vi "VPA QC Try Get Old File Data.vi"(10 "Path (dialog)":path, 11 "State Data In":T4) -> (3 "State Cluster Out":T4)   [LabVIEW 2013]
uses:
  Controls/VPA QC State Data Cluster.ctl
  Controls/VPA QC General Cluster.ctl
  Controls/VPA QC State Enum.ctl
  Controls/VPA QC Bool Cluster.ctl
  Controls/VPA QC State Data Cluster Ver 4.ctl
panel:
  in  "State Cluster Ver  4":T1
  # "Assembly Checklist"
  # "Assembly Checklist"
  # "Assembly Checklist"
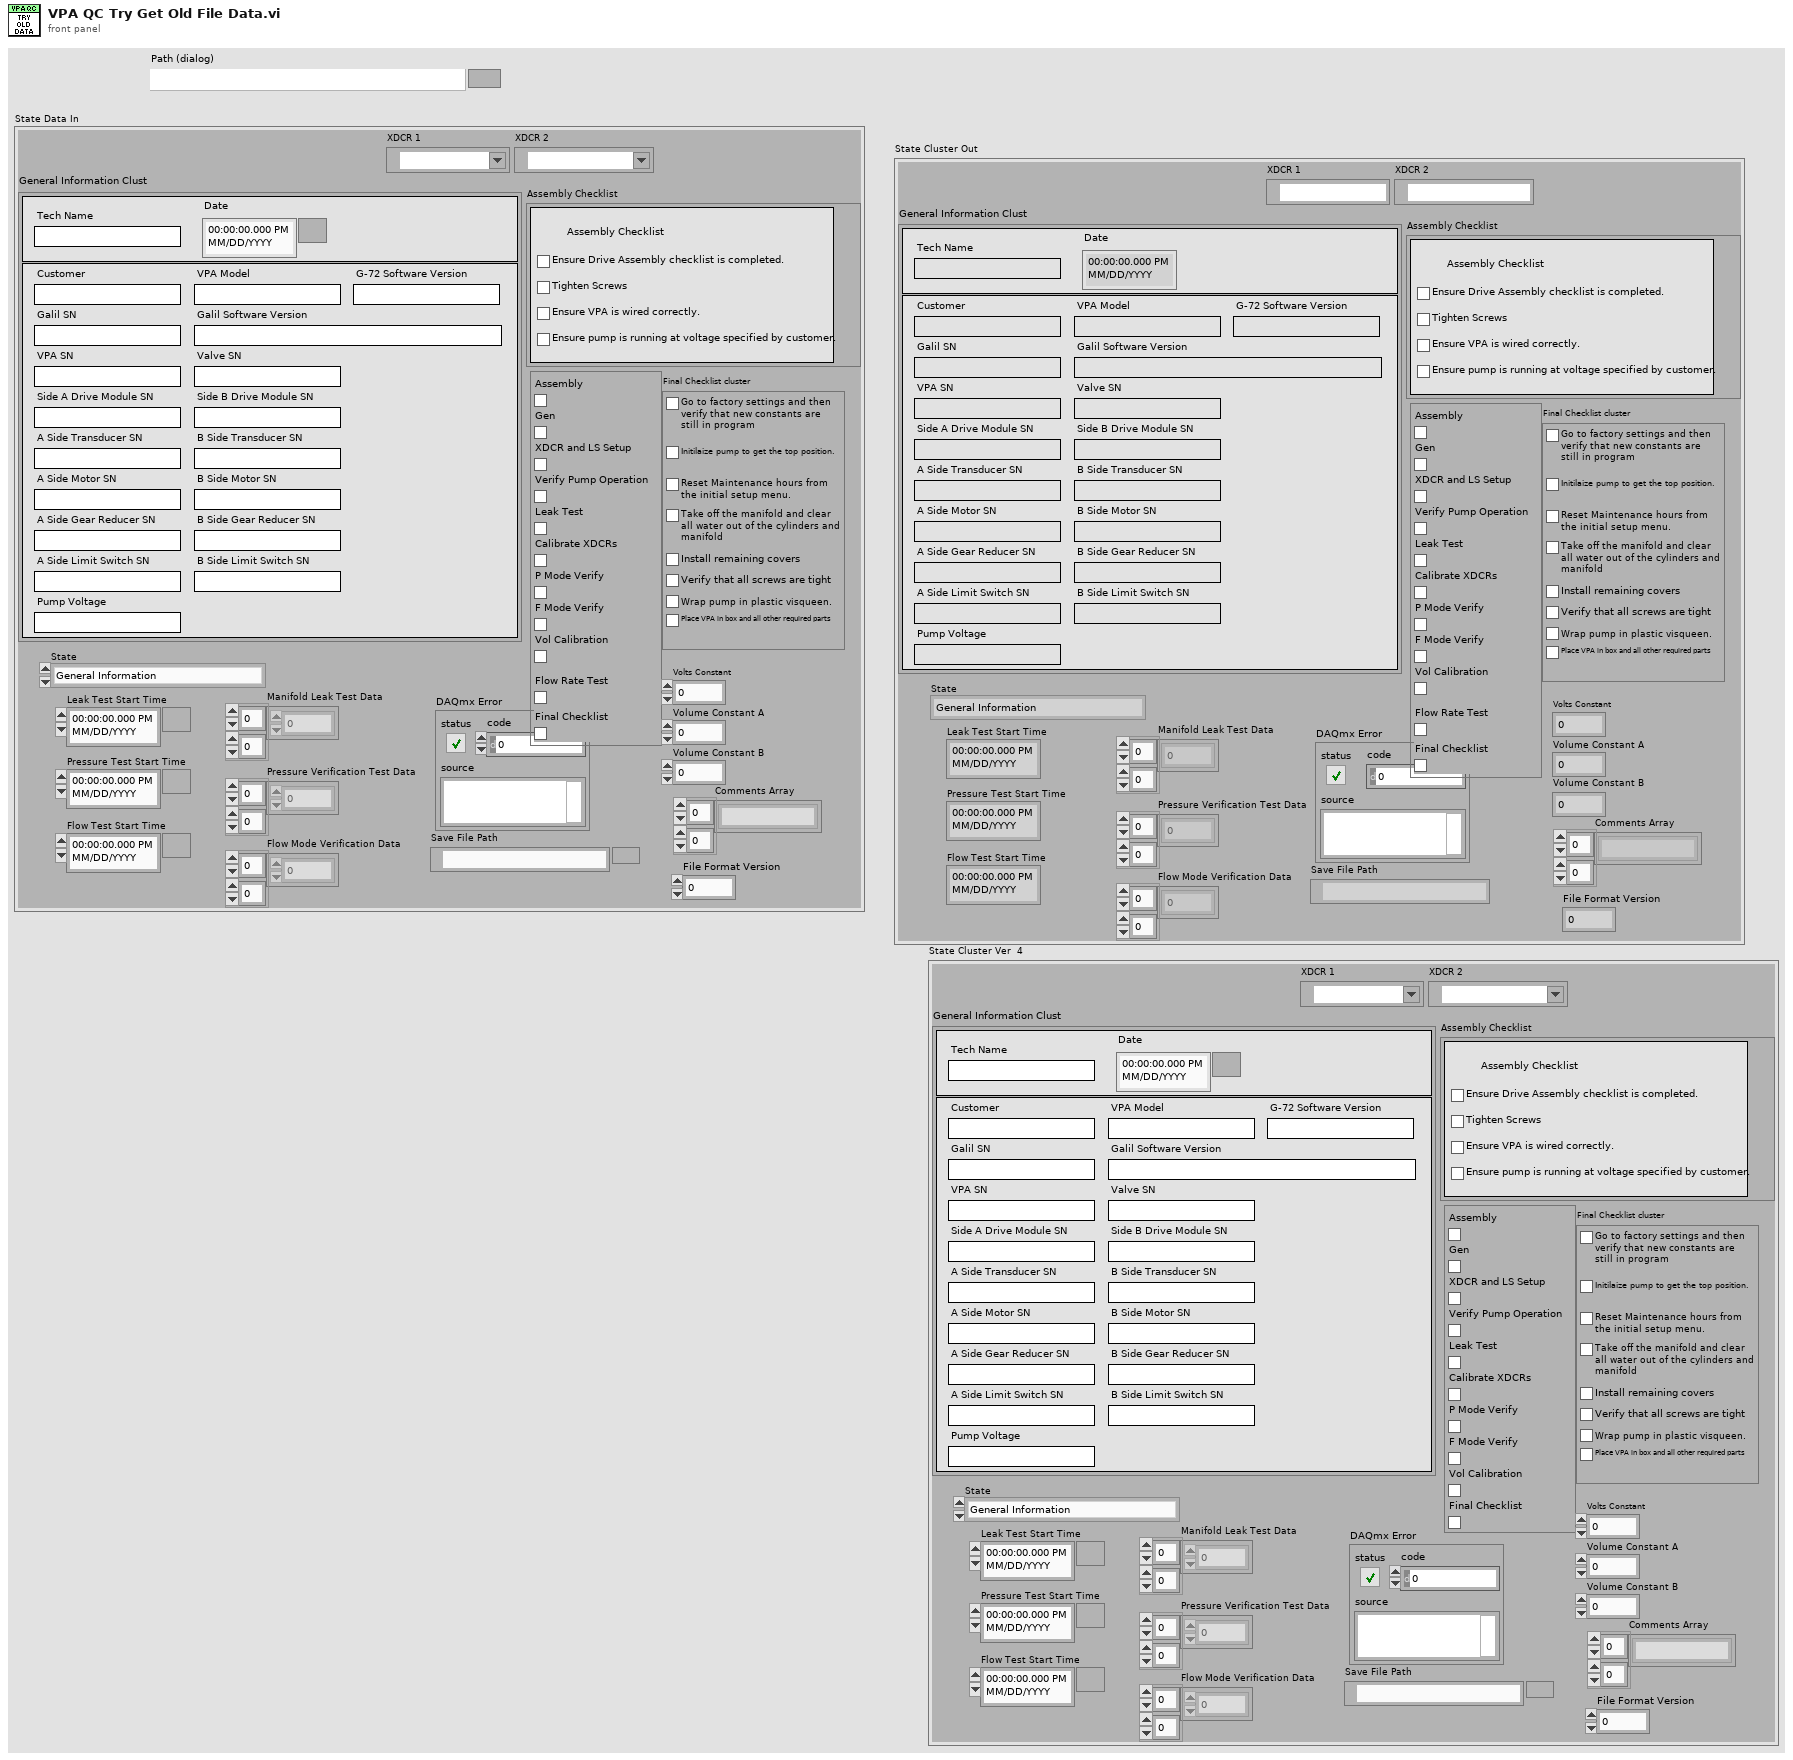
[diagram p1: front panel]
types:
  T1 = typedef "VPA QC State Data Cluster Ver 4.ctl" = cluster{"XDCR 1":tag, "XDCR 2":tag, "General Information Clust":T2, "Assembly Checklist":cluster{"Ensure Drive Assembly checklist is completed.":bool, "Tighten Screws":bool, "Ensure VPA is wired correctly.":bool, "Ensure pump is running at voltage specified by customer.":bool}, "State":T3, "Manifold Leak Test Data":dbl[][], "Pressure Verification Test Data":dbl[][], "Flow Mode Verification Data":dbl[][], "DAQmx Error":errorcluster, "Bool Cluster":cluster{"Assembly":bool, "Gen":bool, "XDCR and LS Setup":bool, "Verify Pump Operation":bool, "Leak Test":bool, "Calibrate XDCRs":bool, "P Mode Verify":bool, "F Mode Verify":bool, "Vol Calibration":bool, "Final Checklist":bool}, "Leak Test Start Time":timestamp, "Pressure Test Start Time":timestamp, "Flow Test Start Time":timestamp, "Final Checklist cluster":cluster{"Check Fact Rest":bool, "Initialize Pump":bool, "Maintenance Hours":bool, "Clean Water Out":bool, "Covers":bool, "Screws":bool, "Wrap":bool, "Box":bool}, "Volts Constant":dbl, "Volume Constant A":dbl, "Volume Constant B":dbl, "Save File Path":path, "Comments Array":string[][], "File Format Version":u16}
  T2 = typedef "VPA QC General Cluster.ctl" = cluster{"Tech Name":string, "Date":timestamp, "Customer":string, "VPA Model":string, "G-72 Software Version":string, "Galil SN":string, "Galil Software Version":string, "VPA SN":string, "Valve SN":string, "Side A Drive Module SN":string, "Side B Drive Module SN":string, "A Side Transducer SN":string, "B Side Transducer SN":string, "A Side Motor SN":string, "B Side Motor SN":string, "A Side Gear Reducer SN":string, "B Side Gear Reducer SN":string, "A Side Limit Switch SN":string, "B Side Limit Switch SN":string, "Pump Voltage":string}
  T3 = typedef "VPA QC State Enum.ctl" = enum16{"General Information", "XDCR and LS Check", "Check Pump Function", "Manifold/Cylinder Leak Test", "Exit"}
  T4 = typedef "VPA QC State Data Cluster.ctl" = cluster{"XDCR 1":tag, "XDCR 2":tag, "General Information Clust":T2, "Assembly Checklist":cluster{"Ensure Drive Assembly checklist is completed.":bool, "Tighten Screws":bool, "Ensure VPA is wired correctly.":bool, "Ensure pump is running at voltage specified by customer.":bool}, "State":T3, "Manifold Leak Test Data":dbl[][], "Pressure Verification Test Data":dbl[][], "Flow Mode Verification Data":dbl[][], "DAQmx Error":errorcluster, "Bool Cluster":T5, "Leak Test Start Time":timestamp, "Pressure Test Start Time":timestamp, "Flow Test Start Time":timestamp, "Final Checklist cluster":cluster{"Check Fact Rest":bool, "Initialize Pump":bool, "Maintenance Hours":bool, "Clean Water Out":bool, "Covers":bool, "Screws":bool, "Wrap":bool, "Box":bool}, "Volts Constant":dbl, "Volume Constant A":dbl, "Volume Constant B":dbl, "Save File Path":path, "Comments Array":string[][], "File Format Version":u16}
  T5 = typedef "VPA QC Bool Cluster.ctl" = cluster{"Assembly":bool, "Gen":bool, "XDCR and LS Setup":bool, "Verify Pump Operation":bool, "Leak Test":bool, "Calibrate XDCRs":bool, "P Mode Verify":bool, "F Mode Verify":bool, "Vol Calibration":bool, "Flow Rate Test":bool, "Final Checklist":bool}
  T6 = cluster{"Ensure Drive Assembly checklist is completed.":bool, "Tighten Screws":bool, "Ensure VPA is wired correctly.":bool, "Ensure pump is running at voltage specified by customer.":bool}
  T7 = cluster{"Assembly":bool, "Gen":bool, "XDCR and LS Setup":bool, "Verify Pump Operation":bool, "Leak Test":bool, "Calibrate XDCRs":bool, "P Mode Verify":bool, "F Mode Verify":bool, "Vol Calibration":bool, "Final Checklist":bool}
  T8 = cluster{"Check Fact Rest":bool, "Initialize Pump":bool, "Maintenance Hours":bool, "Clean Water Out":bool, "Covers":bool, "Screws":bool, "Wrap":bool, "Box":bool}
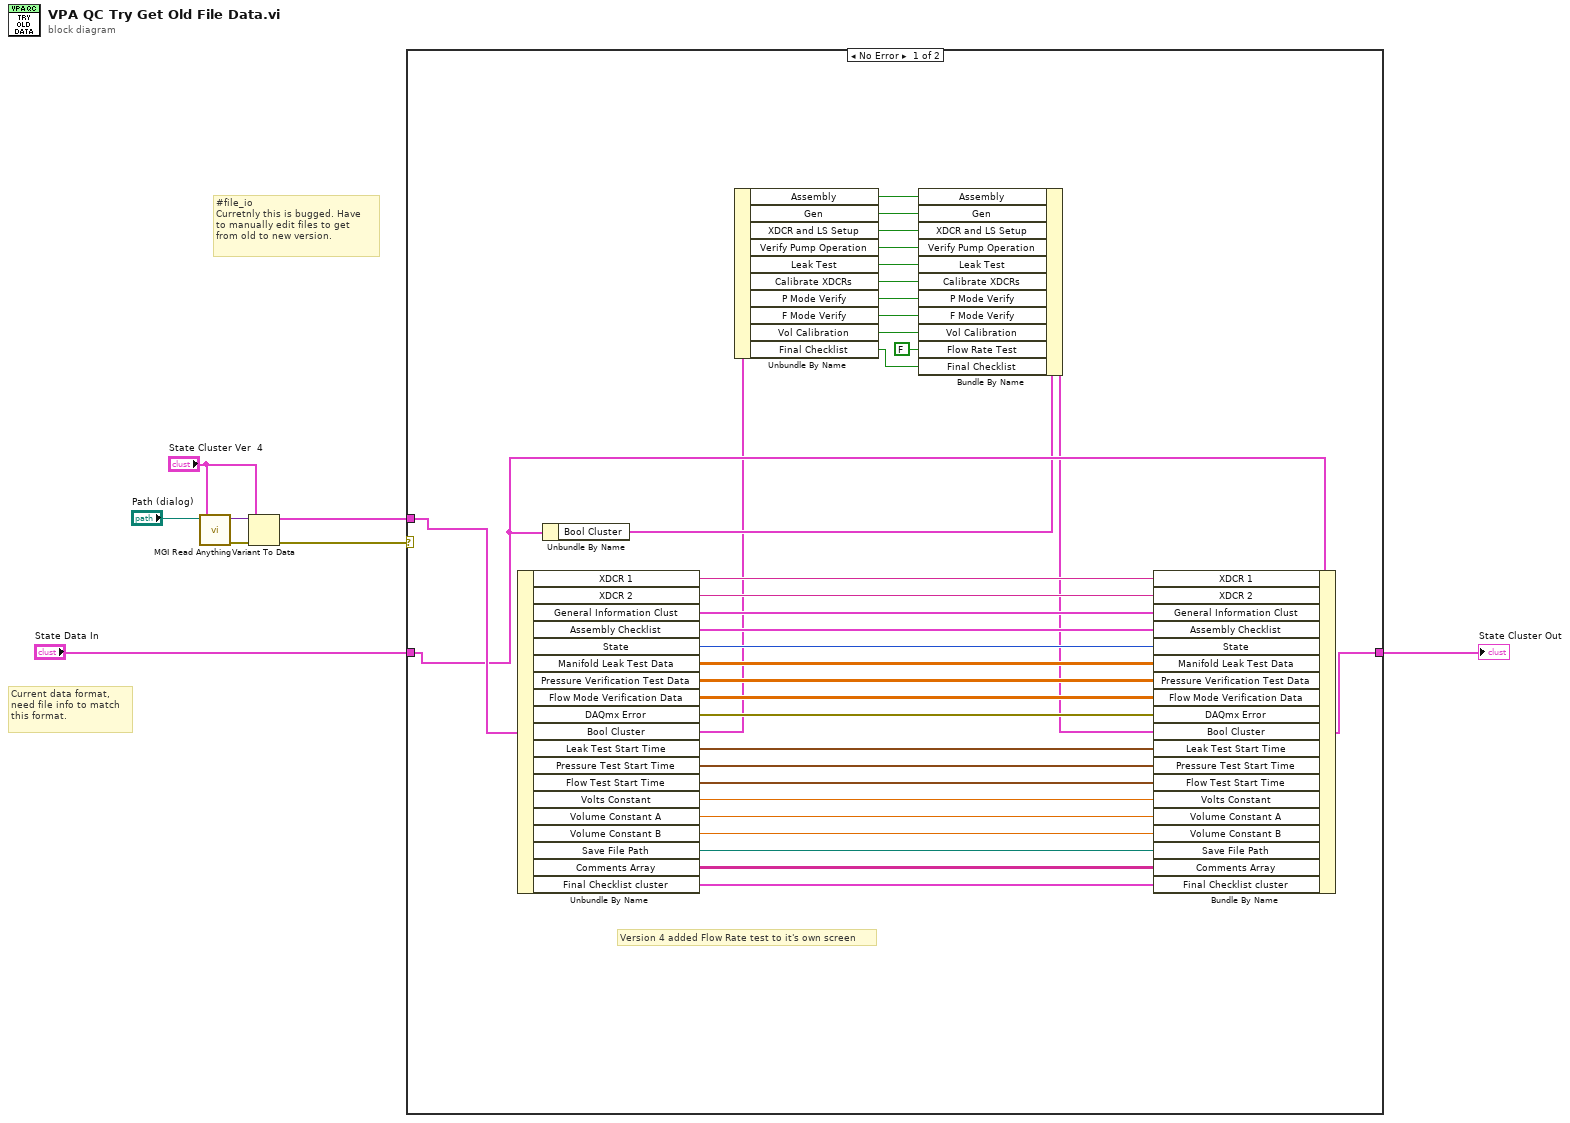
[diagram p0: block diagram]
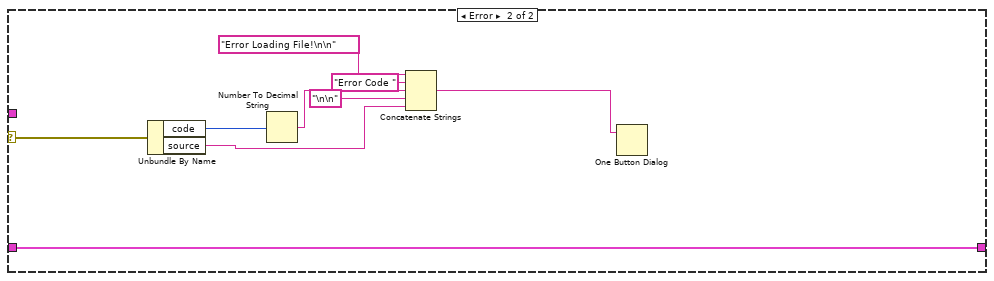
[diagram p2: hidden frame]
diagram:
  # "#file_io\nCurretnly this is bugged. Have \nto manually edit files to get \nfrom old to new version."
  # "Current data format,\nneed file info to match\nthis format."
  n1 = call <userlib>:"MGI Read Anything.vi"("Type of Anything"="State Cluster Ver  4", "Path (dialog)"="Path (dialog)") -> ("Error Out"=w6:errorcluster, "Anything"=w5:variant)  [unwired: 6 in, 2 out]
  n2 = Variant To Data(error in=w6, type="State Cluster Ver  4", Variant=w5) -> (data=w2:T1, error out=w1:errorcluster)
  n3 = case shown="No Error" w1 {
    selector: w1 -> [_ w45]
    tunnel: w2 -> [w28 _]
    tunnel: "State Data In" -> [w25 w44]
    tunnel: [w27 w44] -> w8
    frame No Error {
      # "Version 4 added Flow Rate test to it's own screen"
      n4 = Unbundle By Name(w28) -> ("XDCR 1"=w43:tag, "XDCR 2"=w42:tag, "General Information Clust"=w26:T2, "Assembly Checklist"=w41:T6, "State"=w40:T3, "Manifold Leak Test Data"=w39:dbl[][], "Pressure Verification Test Data"=w38:dbl[][], "Flow Mode Verification Data"=w37:dbl[][], "DAQmx Error"=w36:errorcluster, "Bool Cluster"=w23:T7, "Leak Test Start Time"=w35:timestamp, "Pressure Test Start Time"=w34:timestamp, "Flow Test Start Time"=w33:timestamp, "Volts Constant"=w32:dbl, "Volume Constant A"=w31:dbl, "Volume Constant B"=w30:dbl, "Save File Path"=w29:path, "Comments Array"=w10:string[][], "Final Checklist cluster"=w9:T8)
      n5 = Unbundle By Name(w25) -> ("Bool Cluster"=w24:T5)
      n6 = Unbundle By Name(w23) -> ("Assembly"=w22:bool, "Gen"=w21:bool, "XDCR and LS Setup"=w20:bool, "Verify Pump Operation"=w19:bool, "Leak Test"=w18:bool, "Calibrate XDCRs"=w17:bool, "P Mode Verify"=w16:bool, "F Mode Verify"=w15:bool, "Vol Calibration"=w14:bool, "Final Checklist"=w13:bool)
      n7 = Bundle By Name(cluster=w24, "Assembly"=w22, "Gen"=w21, "XDCR and LS Setup"=w20, "Verify Pump Operation"=w19, "Leak Test"=w18, "Calibrate XDCRs"=w17, "P Mode Verify"=w16, "F Mode Verify"=w15, "Vol Calibration"=w14, "Flow Rate Test"=FALSE, "Final Checklist"=w13) -> (w11:T5)
      n8 = Bundle By Name(cluster=w25, "XDCR 1"=w43, "XDCR 2"=w42, "General Information Clust"=w26, "Assembly Checklist"=w41, "State"=w40, "Manifold Leak Test Data"=w39, "Pressure Verification Test Data"=w38, "Flow Mode Verification Data"=w37, "DAQmx Error"=w36, "Bool Cluster"=w11, "Leak Test Start Time"=w35, "Pressure Test Start Time"=w34, "Flow Test Start Time"=w33, "Volts Constant"=w32, "Volume Constant A"=w31, "Volume Constant B"=w30, "Save File Path"=w29, "Comments Array"=w10, "Final Checklist cluster"=w9) -> (w27:T4)
    }
    frame Error {
      n9 = Unbundle By Name(w45) -> ("code"=w52:i32, "source"=w47:string)
      n10 = Number To Decimal String(number=w52) -> (decimal integer string=w49:string)  [unwired: 1 in]
      n11 = Concatenate Strings("Error Loading File!\n\n" ("message"), "Error Code " ("string"), w49, "\n\n" ("string"), w47) -> (w46:string)
      n12 = One Button Dialog(message=w46) -> ()  [unwired: 1 in, 1 out]
    }
  }
  "State Cluster Out" <- w8
